vi "String Array To String.vi"(10 "Array - String":string[](array[string])) -> (1 "length":i32, 2 "Output string":string)   [LabVIEW 2014]
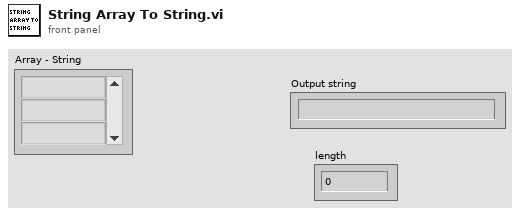
[diagram p1: front panel]
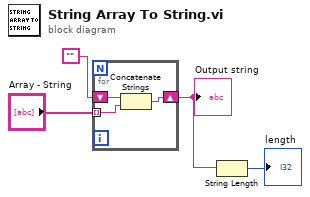
[diagram p0: block diagram]
diagram:
  n1 = for {
    tunnel: "Array - String" -> [w6] mode=indexing
    shift-right: [w5] -> w2
    shift-left: "" -> [w7]
    n2 = Concatenate Strings(w7, w6) -> (w5:string)
  }
  "Output string" <- w2
  n3 = String Length(string=w2) -> (length=→"length":i32)
